vi "SetTriggerLevel.vi"(2 "error in (no error)":errorcluster, 3 "Trigger In Selection":u8(ring) items=["Value", "Minimum", "Maximum", "Default"], 4 "Trigger In Threshold (V)":dbl=1.0, 5 "VISA resource name":refnum<visa-resource-name>) -> (0 "error out":errorcluster, 1 "VISA resource name out":refnum<visa-resource-name>)   [LabVIEW 2020, in "Active Technologies AWG3000.lvlib"]
uses:
  Active Technologies AWG3000.lvlib
panel:
  out "VISA WRITE":string
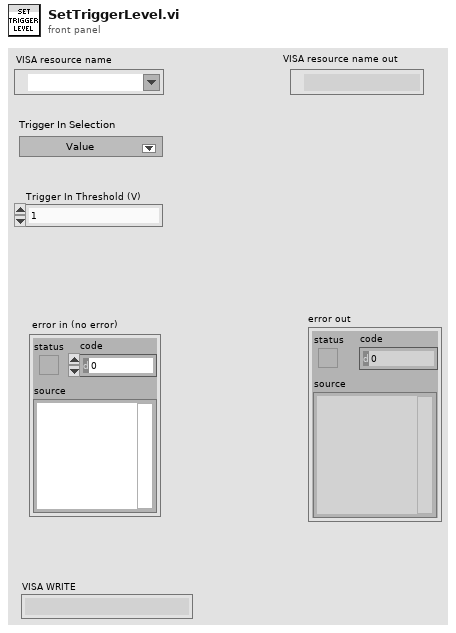
[diagram p1: front panel]
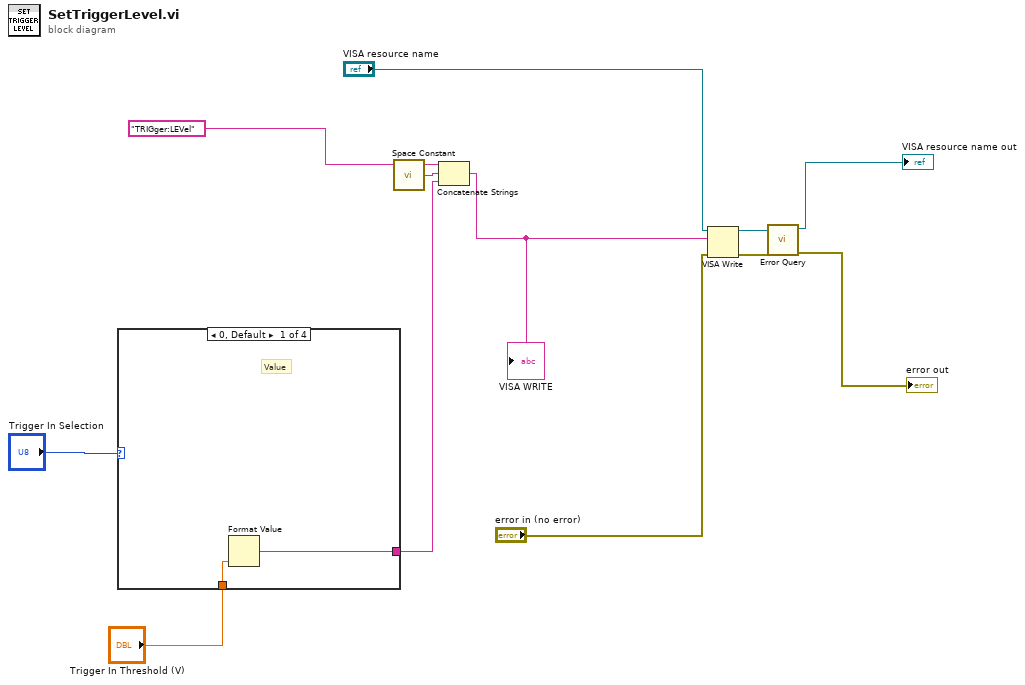
[diagram p0: block diagram]
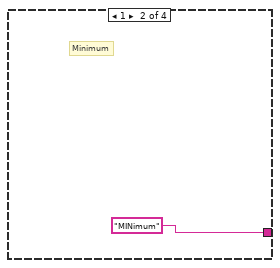
[diagram p2: hidden frame]
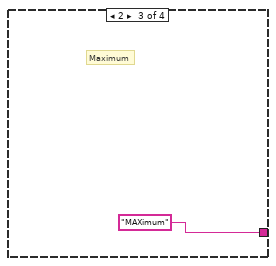
[diagram p3: hidden frame]
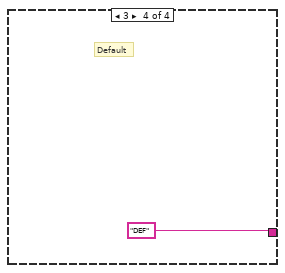
[diagram p4: hidden frame]
diagram:
  n1 = case shown="0, Default" "Trigger In Selection" {
    tunnel: "Trigger In Threshold (V)" -> [w14 _ _ _]
    tunnel: [w13 "MINimum" "MAXimum" "DEF"] -> w3
    frame 0, Default {
      # "Value"
      n2 = Format Value(value (0)=w14) -> (output string=w13:string)  [unwired: 2 in]
    }
    frame 1 {
      # "Minimum"
    }
    frame 2 {
      # "Maximum"
    }
    frame 3 {
      # "Default"
    }
  }
  n3 = call <vilib>:"Space Constant.vi"() -> ("String"=w5:string)
  n4 = Concatenate Strings("TRIGger:LEVel" ("write buffer"), w5, w3) -> (w2:string)
  "VISA WRITE" <- w2
  n5 = VISA Write(VISA resource name="VISA resource name", write buffer=w2, error in (no error)="error in (no error)") -> (VISA resource name out=w10:refnum<visa-resource-name>, error out=w9:errorcluster)  [unwired: 1 out]
  n6 = call "Error Query.vi"("error in (no error)"=w9, "VISA resource name"=w10) -> ("error out"=→"error out":errorcluster, "VISA resource name out"=→"VISA resource name out":refnum<visa-resource-name>)  [unwired: 6 in, 2 out]
